vi "ramp array.vi"(2 "ramp mode":T1(ring), 3 "initialize":cluster{"init values":dbl[], "reset":bool}, 4 "max change/s":dbl, 5 "setpoint":dbl[](array[slide]) scale=-1.0..1.0) -> (0 "seconds elapsed":dbl format="%.2f", 1 "output":dbl[](array[slide]) scale=-1.0..1.0)   [LabVIEW 2009]
doc: "Ramps a value or array of values. In order for the array portion to function properly, it must be initialized (so that it knows how large the array is)"
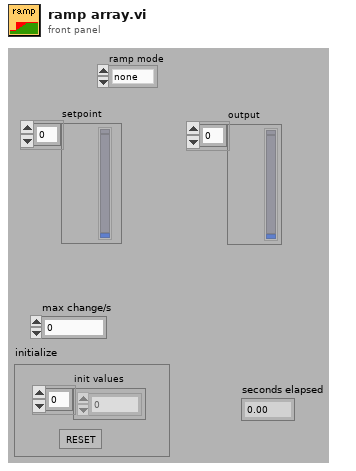
[diagram p1: front panel]
types:
  T1 = enum8{"none", "descel only", "accel only", "both"}
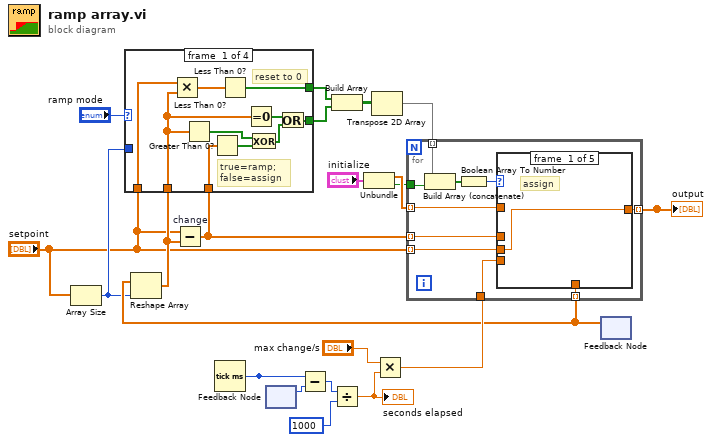
[diagram p0: block diagram]
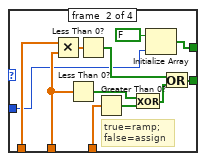
[diagram p2: hidden frame]
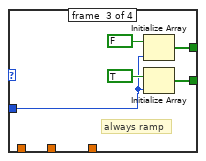
[diagram p3: hidden frame]
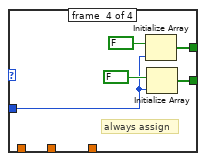
[diagram p4: hidden frame]
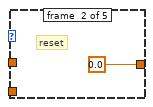
[diagram p5: hidden frame]
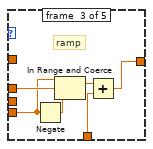
[diagram p6: hidden frame]
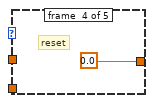
[diagram p7: hidden frame]
diagram:
  n1 = Array Size(array="setpoint") -> (size(s)=w12:i32)
  n2 = Tick Count (ms)() -> (millisecond timer value=w20:u32)
  n3 = feedback #1() -> (w21:u32)  [unwired: 1 in]
  n4 = Subtract(x=w20, y=w21) -> (x-y=w3:u32)
  n5 = Divide(x=w3, y=u32 1000) -> (x/y=w2:dbl)
  "seconds elapsed" <- w2
  n6 = Unbundle("initialize") -> ("init values"=w18:dbl[], "reset"=w15:bool)
  n7 = Multiply(x="max change/s", y=w2) -> (x*y=w17:dbl)
  n8 = feedback #2() -> (w14:dbl[])  [unwired: 1 in]
  n9 = Reshape Array(w14, w12) -> (w6:dbl[])
  n10 = Subtract "change"(x="setpoint", y=w6) -> (x-y=w7:dbl[])
  n11 = case shown="\"none\"" "ramp mode" {
    tunnel: w7 -> [w31 w43 _ _]
    tunnel: "setpoint" -> [w30 w42 _ _]
    tunnel: [w29 w33 w45 w50] -> w10
    tunnel: w6 -> [w28 w41 _ _]
    tunnel: [w27 w40 w44 w53] -> w11
    tunnel: w12 -> [_ w32 w46 w49]
    frame #0 {
      # "reset to 0"
      # "true=ramp;\nfalse=assign"
      n12 = Multiply(x=w30, y=w28) -> (x*y=w24:dbl[])
      n13 = Less Than 0?(x=w28) -> (x < 0?=w25:bool[])
      n14 = Greater Than 0?(x=w31) -> (x > 0?=w26:bool[])
      n15 = Less Than 0?(x=w24) -> (x < 0?=w29:bool[])
      n16 = Equal To 0?(x=w28) -> (x = 0?=w23:bool[])
      n17 = Exclusive Or(1:w26, 2:w25) -> (0:w22:bool[])
      n18 = Or(x=w23, y=w22) -> (x .or. y?=w27:bool[])
    }
    frame #1 {
      # "true=ramp;\nfalse=assign"
      n19 = Multiply(x=w42, y=w41) -> (x*y=w37:dbl[])
      n20 = Less Than 0?(x=w41) -> (x < 0?=w38:bool[])
      n21 = Less Than 0?(x=w37) -> (x < 0?=w35:bool[])
      n22 = Greater Than 0?(x=w43) -> (x > 0?=w39:bool[])
      n23 = Exclusive Or(1:w39, 2:w38) -> (0:w36:bool[])
      n24 = Initialize Array(FALSE, w32) -> (w33:bool[])
      n25 = Or(x=w35, y=w36) -> (x .or. y?=w40:bool[])
    }
    frame #2 {
      # "always ramp"
      n26 = Initialize Array(FALSE, w46) -> (w45:bool[])
      n27 = Initialize Array(TRUE, w46) -> (w44:bool[])
    }
    frame #3 {
      # "always assign"
      n28 = Initialize Array(FALSE, w49) -> (w50:bool[])
      n29 = Initialize Array(FALSE, w49) -> (w53:bool[])
    }
  }
  n30 = Build Array(w10, w11) -> (w9:bool[][])
  n31 = Transpose 2D Array(2D array=w9) -> (transposed array=w8:bool[][])
  n32 = for {
    tunnel: w18 -> [w63] mode=indexing
    tunnel: w7 -> [w62] mode=indexing
    tunnel: w17 -> [w61]
    tunnel: w14 -> [w60] mode=indexing
    tunnel: "setpoint" -> [w59] mode=indexing
    tunnel: [w58] -> w16 mode=indexing
    tunnel: w8 -> [w57] mode=indexing
    tunnel: w15 -> [w56]
    n33 = Build Array (concatenate)(w57, w56) -> (w55:bool[])
    n34 = Boolean Array To Number(Boolean array=w55) -> (number=w54:u32)
    n35 = case shown="0, Default" w54 {
      tunnel: [w64 0.0 ("value") w68 0.0 w73] -> w58
      tunnel: w63 -> [_ _ _ _ w73]
      tunnel: w60 -> [_ _ w69 _ _]
      tunnel: w62 -> [_ _ w67 _ _]
      tunnel: w61 -> [_ _ w66 _ _]
      tunnel: w59 -> [w64 _ _ _ _]
      frame #0 {
        # "assign"
      }
      frame #1 {
        # "reset"
      }
      frame #2 {
        # "ramp"
        n36 = Negate(x=w66) -> (-x=w71:dbl)
        n37 = In Range and Coerce(upper limit=w66, x=w67, lower limit=w71) -> (coerced(x)=w70:dbl)  [unwired: 1 out]
        n38 = Add(x=w70, y=w69) -> (x+y=w68:dbl)
      }
      frame #3 {
        # "reset"
      }
      frame #4 {
        # "initialize"
      }
    }
  }
  "output" <- w16
